vi "read field - fast.vi"(8 "error in (no error)":errorcluster, 11 "VISA resource name":refnum<visa-resource-name>="GPIB0::2::INSTR") -> (0 "error out":errorcluster, 2 "Current field (T)":dbl[unit], 3 "VISA resource name out":refnum<visa-resource-name>)   [LabVIEW 2009, in "Varian Magnet.lvclass"]
uses:
  Varian Magnet.lvclass
  Fluke Multimeter/Fluke 8840/Fluke 8840.lvlib
panel:
  out "unit":string
  out "measurement":dbl format="%^.6e"
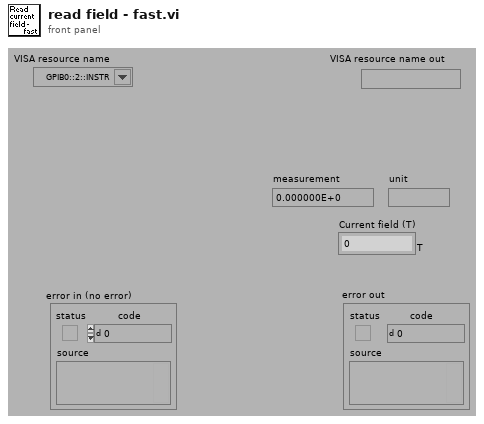
[diagram p1: front panel]
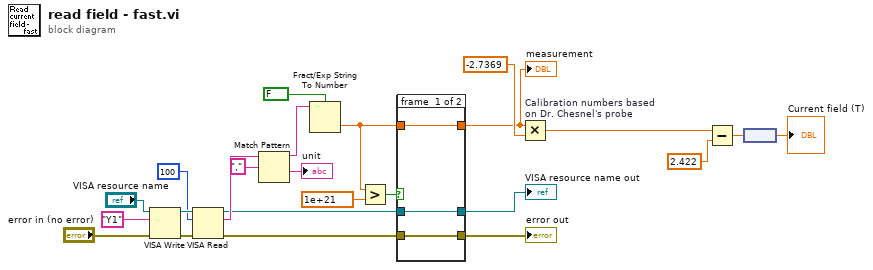
[diagram p0: block diagram]
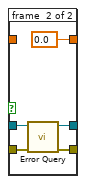
[diagram p2: hidden frame]
diagram:
  n1 = VISA Write(VISA resource name="VISA resource name", write buffer="Y1", error in (no error)="error in (no error)") -> (VISA resource name out=w21:refnum<visa-resource-name>, error out=w22:errorcluster)  [unwired: 1 out]
  n2 = VISA Read(VISA resource name=w21, byte count=100, error in (no error)=w22) -> (VISA resource name out=w10:refnum<visa-resource-name>, read buffer=w16:string, error out=w11:errorcluster)  [unwired: 1 out]
  n3 = Match Pattern(string=w16, regular expression=",") -> (before substring=w18:string, after substring=→"unit":string)  [unwired: 3 out]
  n4 = Fract/Exp String To Number(use system decimal point (T)=FALSE, string=w18) -> (number=w9:dbl)  [unwired: 3 out]
  n5 = Greater?(x=w9, y=1e+21) -> (0:w14:bool)
  n6 = case shown="True" w14 {
    tunnel: [w27 0.0] -> w1
    tunnel: [w26 w31] -> w13
    tunnel: [w25 w30] -> w12
    tunnel: w11 -> [w25 w29]
    tunnel: w10 -> [w26 w28]
    tunnel: w9 -> [w27 _]
    frame #0 {
    }
    frame #1 {
      n7 = call "Error Query.vi"("error in (no error)"=w29, "VISA resource name"=w28) -> ("error out"=w30:errorcluster, "VISA resource name out"=w31:refnum<visa-resource-name>)  [unwired: 1 in, 7 out]
    }
  }
  "error out" <- w12
  "VISA resource name out" <- w13
  "measurement" <- w1
  n8 = Multiply "Calibration numbers based\non Dr. Chesnel's probe"(x=w1, y=-2.7369) -> (x*y=w5:dbl)
  n9 = Subtract(x=w5, y=2.422 ("x")) -> (x-y=w4:dbl)
  n10 = node(w4) -> (→"Current field (T)":dbl[unit])
